vi "CRYAttack and Release.vi"(4 "Sine waves":T1(array[cluster]), 5 "Attack":sgl[](array[numeric]), 6 "Search range":string[](array[string]), 7 "% recovery":dbl=0.02 format="%.2f", 8 "All points":bool, 9 "Sampling rate":dbl format="%.2f", 10 "Attack? (T)":bool=TRUE, 11 "Data in":T2={"Name"="", "Curve"=[], "X data"=1, "Y data"=1, "Z data"=1, "X axis"=0, "Y axis"=1, "Z axis"=1, "X unit"="Hz", "Y unit"="", "Z unit"="deg.", "X dB ref"=1.0, "Y dB ref"=1.0, "Z dB ref"=1.0, "single val"=FALSE, "protected"=FALSE, "display X"=TRUE, "display Y"=TRUE, "display Z"=TRUE, "Test Info"="", "Step No."=0, "Plot Settings"={"Color"=0, "Interpolation"=0, "Point Style"=0, "Line Style"=0, "Point Color"=0, "Line Width"=0, "Bar Plot Style"=0, "Fill To"=0}, "AutoProtect"=FALSE} {"Z data" items=["dB", "Lin"]; "X data" items=["dB", "Lin"]; "Y data" items=["dB", "Lin"]; "Z dB ref" format="%.1f"; "Z axis" items=["Log", "Lin"]; "X dB ref" format="%.1f"; "X axis" items=["Log", "Lin"]; "Y axis" items=["Log", "Lin"]; "Y dB ref" format="%.1f"; "Curve"."z" format="%.2f"; "Curve"."y" format="%.2f"; "Curve"."x" format="%.2f"}) -> (1 "dy":dbl, 2 "Envelope":dbl[](array[numeric]) format="%.2f", 3 "Attack or release time":dbl format="%.2f")   [LabVIEW 2013]
uses:
  Typedef Control/CRYData Cluster.ctl
  <vilib>/Analysis/2dsp.llb/Decimate (single shot, DBL).vi
  <vilib>/Analysis/3filter.llb/Bessel Filter (DBL).vi
  <vilib>/Analysis/NI_AALPro.lvlib
  <vilib>/Analysis/NI_AALBase.lvlib
panel:
  out "dy 2":dbl
  out "Waveform Graph 2":waveform(dbl)(graph)
  out "Waveform Graph":waveform(dbl)(graph)
  in  "Discard cycles right":i32
  in  "search for attack/release starting point?":bool=TRUE
  in  "I donot know?":bool
  in  "BP filtering":bool=TRUE
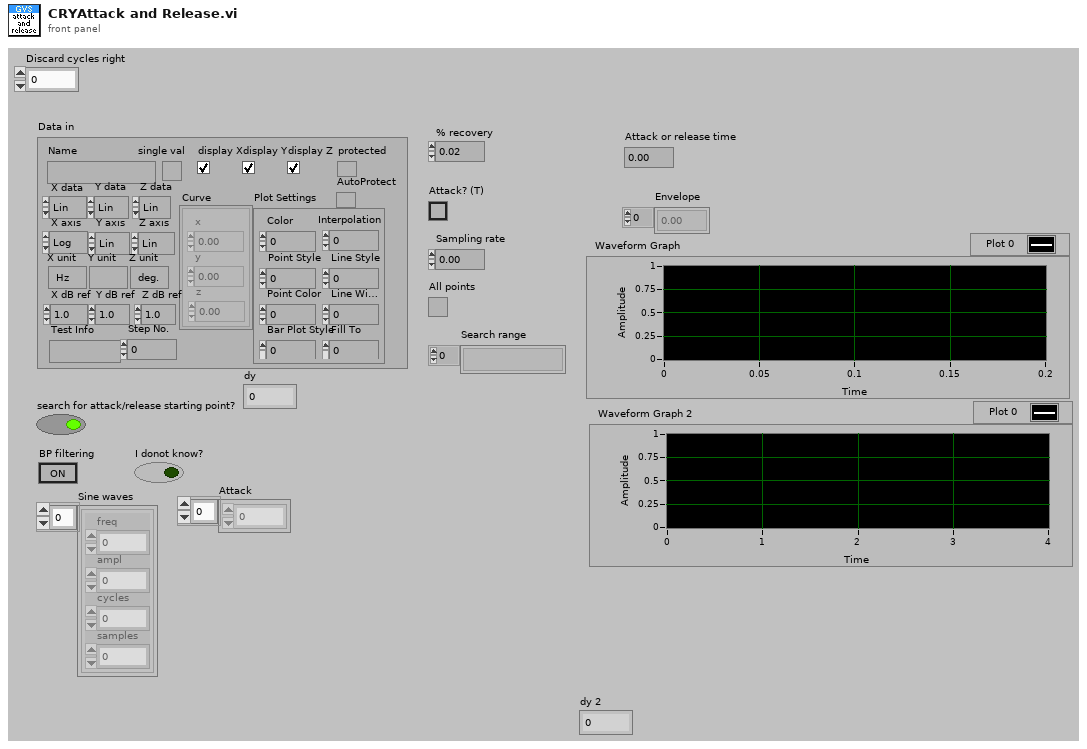
[diagram p1: front panel]
types:
  T1 = cluster{"freq":dbl, "ampl":dbl, "cycles":dbl, "samples":i32}[]
  T2 = typedef "CRYData Cluster.ctl" = cluster{"Name":string, "Curve":cluster{"x":dbl, "y":dbl, "z":dbl}[], "X data":u16, "Y data":u16, "Z data":u16, "X axis":u16, "Y axis":u16, "Z axis":u16, "X unit":string, "Y unit":string, "Z unit":string, "X dB ref":dbl, "Y dB ref":dbl, "Z dB ref":dbl, "single val":bool, "protected":bool, "display X":bool, "display Y":bool, "display Z":bool, "Test Info":string, "Step No.":i32, "Plot Settings":cluster{"Color":u32, "Interpolation":u8, "Point Style":u8, "Line Style":u8, "Point Color":u32, "Line Width":u8, "Bar Plot Style":u8, "Fill To":i16}, "AutoProtect":bool}
  T3 = cluster{"freq":dbl, "ampl":dbl, "cycles":dbl, "samples":i32}
  T4 = enum32{"Lowpass", "Highpass", "Bandpass", "Bandstop"}
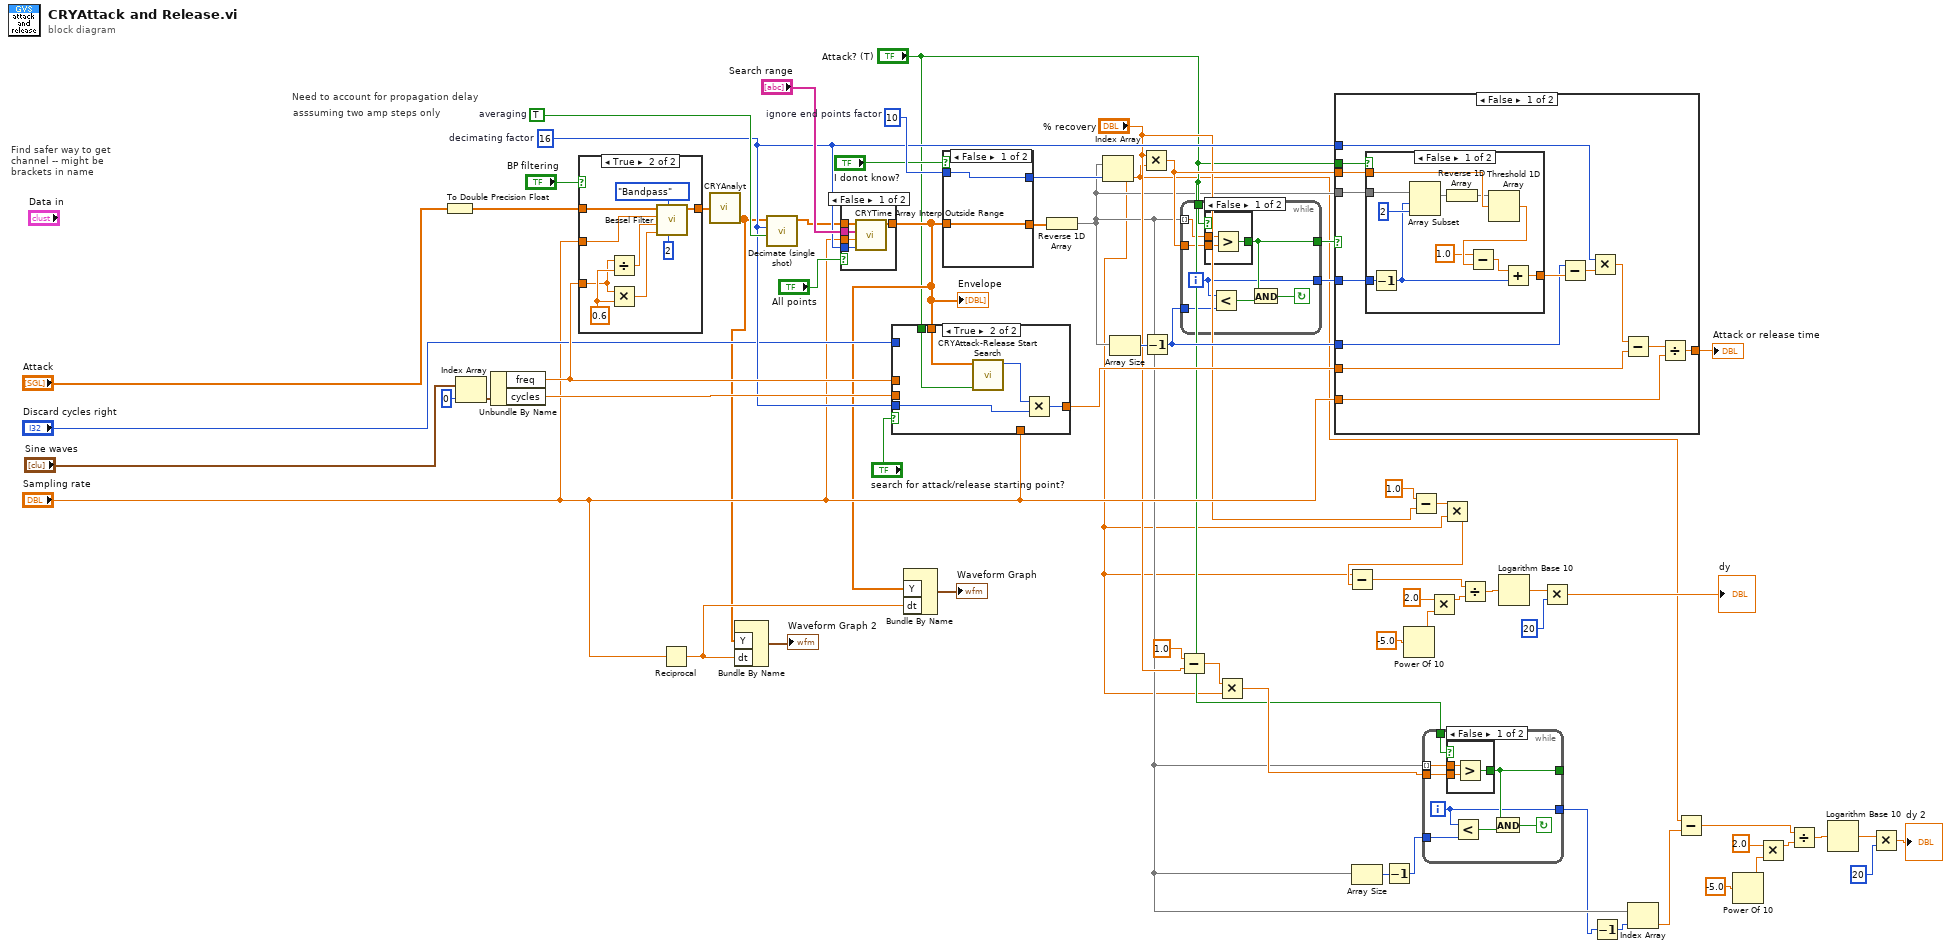
[diagram p0: block diagram]
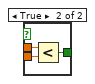
[diagram p2: hidden frame]
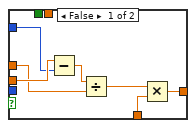
[diagram p3: hidden frame]
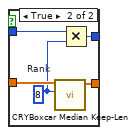
[diagram p5: hidden frame]
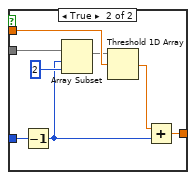
[diagram p7: hidden frame]
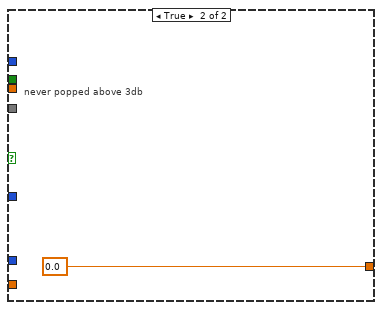
[diagram p8: hidden frame]
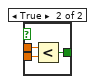
[diagram p9: hidden frame]
diagram:
  w57 = 10  # ignore end points factor
  w66 = TRUE  # averaging
  w48 = 16  # decimating factor
  # "Need to account for propagation delay"
  # "asssuming two amp steps only"
  # "Find safer way to get channel -- might be brackets in name"
  n1 = To Double Precision Float(number="Attack") -> (double precision float=w52:dbl[])
  n2 = Index Array(array="Sine waves", index=0 ("Index")) -> (element=w60:T3)
  n3 = Unbundle By Name(w60) -> ("freq"=w55:dbl, "cycles"=w56:dbl)
  n4 = case shown="True" "BP filtering" {
    tunnel: [w67 w76] -> w42
    tunnel: w52 -> [w67 w71]
    tunnel: w55 -> [_ w70]
    tunnel: "Sampling rate" -> [_ w69]
    frame False {
    }
    frame True {
      w75 = 0.6
      n5 = Divide(x=w70, y=w75) -> (x/y=w74:dbl)
      n6 = Multiply(x=w70, y=w75) -> (x*y=w73:dbl)
      n7 = call-poly <vilib>:"Bessel Filter.vi"("order"=2, "filter type"=T4."Bandpass", "low cutoff freq: fl"=w73, "high cutoff freq: fh"=w74, "sampling freq: fs"=w69, "X"=w71) -> ("Filtered X"=w76:dbl[])  [unwired: 1 in, 2 out]
    }
  }
  n8 = Reciprocal(x="Sampling rate") -> (1/x=w40:dbl)
  n9 = call "CRYAnalyt.vi"("Input"=w42) -> ("Magn"=w37:dbl[])  [unwired: 4 out]
  n10 = Bundle By Name("Y"=w37, "dt"=w40) -> (→"Waveform Graph 2":waveform(dbl))  [unwired: 1 in]
  n11 = call-poly <vilib>:"Decimate (single shot).vi"("averaging"=w66, "decimating factor"=w48, "X"=w37) -> ("Decimated Array"=w38:dbl[])  [unwired: 8 out]
  n12 = case shown="False" "All points" {
    tunnel: w38 -> [w81 w82]
    tunnel: [w80 w82] -> w41
    tunnel: "Search range" -> [w79 _]
    tunnel: "Sampling rate" -> [w78 _]
    tunnel: w48 -> [w77 _]
    frame False {
      n13 = call "CRYTime Array Interp Outside Range.vi"("Decimating factor"=w77, "Sampling rate"=w78, "Search range (ms)"=w79, "Points in time"=w81) -> ("Processed points in time"=w80:dbl[])  [unwired: 7 out]
    }
    frame True {
    }
  }
  "Envelope" <- w41
  n14 = case shown="True" "search for attack/release starting point?" {
    tunnel: [w88 w90] -> w59
    tunnel: w56 -> [w87 _]
    tunnel: "Discard cycles right" -> [w85 _]
    tunnel: w55 -> [w84 _]
    tunnel: "Sampling rate" -> [w83 _]
    tunnel: w41 -> [_ w94]
    tunnel: "Attack? (T)" -> [_ w93]
    tunnel: w48 -> [_ w92]
    frame False {
      n15 = Subtract(x=w87, y=w85) -> (x-y=w86:dbl)
      n16 = Divide(x=w86, y=w84) -> (x/y=w89:dbl)
      n17 = Multiply(x=w89, y=w83) -> (x*y=w88:dbl)
    }
    frame True {
      n18 = call "CRYAttack-Release Start Search.vi"("Attack? (T)"=w93, "Time data in"=w94) -> ("Pulse start index"=w91:i32)  [unwired: 2 in, 7 out]
      n19 = Multiply(x=w91, y=w92) -> (x*y=w90:i32)
    }
  }
  n20 = Bundle By Name("Y"=w41, "dt"=w40) -> (→"Waveform Graph":waveform(dbl))  [unwired: 1 in]
  n21 = case shown="False" "I donot know?" {
    tunnel: w41 -> [w96 w101]
    tunnel: [w96 w100] -> w58
    tunnel: w57 -> [w95 w98]
    tunnel: [w95 w97] -> w34
    frame False {
    }
    frame True {
      w99 = 8  # Rank
      n22 = call "CRYBoxcar Median Keep-Len.vi"("Rank"=w99, "Measured curve"=w101) -> ("Smoothed curve"=w100:dbl[])  [unwired: 9 out]
      n23 = Multiply(x=w98, y=w99) -> (x*y=w97:i32)
    }
  }
  n24 = Reverse 1D Array(array=w58) -> (reversed array=w13:dbl[])
  n25 = Index Array(array=w13, index=w34) -> (element=w1:dbl)
  n26 = Array Size(array=w13) -> (size(s)=w65:i32)
  n27 = Multiply(x="% recovery", y=w1) -> (x*y=w22:dbl)
  n28 = Decrement(x=w65) -> (x-1=w63:i32)
  n29 = Subtract(x=1.0, y="% recovery") -> (x-y=w16:dbl)
  n30 = while {
    tunnel: w13 -> [w107] mode=indexing
    tunnel: w63 -> [w109]
    tunnel: w22 -> [w108]
    tunnel: [w104] -> w64
    tunnel: [w103] -> w35
    tunnel: "Attack? (T)" -> [w102]
    i -> [w103]
    stop <- w105 continue-if-true
    n31 = case shown="False" w102 {
      tunnel: w108 -> [w111 w115]
      tunnel: w107 -> [w112 w114]
      tunnel: [w110 w113] -> w104
      frame False {
        n32 = Greater?(x=w112, y=w111) -> (0:w110:bool)
      }
      frame True {
        n33 = Less?(x=w114, y=w115) -> (x < y?=w113:bool)
      }
    }
    n34 = Less?(x=w103, y=w109) -> (x < y?=w106:bool)
    n35 = And(x=w104, y=w106) -> (x .and. y?=w105:bool)
  }
  n36 = Multiply(x=w16, y=w1) -> (x*y=w15:dbl)
  n37 = case shown="False" w64 {
    tunnel: w13 -> [w128 _]
    tunnel: w35 -> [w125 _]
    tunnel: w22 -> [w127 _]
    tunnel: w59 -> [w126 _]
    tunnel: w63 -> [w123 _]
    tunnel: "Sampling rate" -> [w122 _]
    tunnel: [w116 0.0] -> w62
    tunnel: w48 -> [w120 _]
    tunnel: "Attack? (T)" -> [w117 _]
    frame False {
      n38 = case shown="False" w117 {
        tunnel: w128 -> [w138 w146]
        tunnel: w127 -> [w137 w145]
        tunnel: w125 -> [w135 w143]
        tunnel: [w134 w141] -> w124
        frame False {
          n39 = Decrement(x=w135) -> (x-1=w133:i32)
          n40 = Array Subset(array=w138, index=w133, length=2 ("Array Length")) -> (w136:dbl[])
          n41 = Reverse 1D Array(array=w136) -> (reversed array=w132:dbl[])
          n42 = Threshold 1D Array(2:w137, 3:w132) -> (0:w131:dbl)  [unwired: 1 out]
          n43 = Subtract(x=1.0, y=w131) -> (x-y=w129:dbl)
          n44 = Add(x=w129, y=w133) -> (x+y=w134:dbl)
        }
        frame True {
          n45 = Decrement(x=w143) -> (x-1=w140:i32)
          n46 = Array Subset(array=w146, index=w140, length=2 ("Array Length")) -> (w144:dbl[])
          n47 = Threshold 1D Array(2:w145, 3:w144) -> (0:w142:dbl)  [unwired: 1 out]
          n48 = Add(x=w142, y=w140) -> (x+y=w141:dbl)
        }
      }
      n49 = Subtract(x=w123, y=w124) -> (x-y=w119:dbl)
      n50 = Multiply(x=w120, y=w119) -> (x*y=w118:dbl)
      n51 = Subtract(x=w118, y=w126) -> (x-y=w121:dbl)
      n52 = Divide(x=w121, y=w122) -> (x/y=w116:dbl)
    }
    frame True {
      # "never popped above 3db"
    }
  }
  "Attack or release time" <- w62
  n53 = Array Size(array=w13) -> (size(s)=w19:i32)
  n54 = Decrement(x=w19) -> (x-1=w20:i32)
  n55 = Power Of 10(x=-5.0) -> (10^x=w29:dbl)
  n56 = Subtract(x=1.0, y="% recovery") -> (x-y=w23:dbl)
  n57 = while {
    tunnel: w20 -> [w156]
    tunnel: w15 -> [w155]
    tunnel: [w152] -> _
    tunnel: [w151] -> w12
    tunnel: "Attack? (T)" -> [w150]
    tunnel: w13 -> [w149] mode=indexing
    i -> [w151]
    stop <- w153 continue-if-true
    n58 = case shown="False" w150 {
      tunnel: w155 -> [w158 w162]
      tunnel: w149 -> [w159 w161]
      tunnel: [w157 w160] -> w152
      frame False {
        n59 = Greater?(x=w159, y=w158) -> (0:w157:bool)
      }
      frame True {
        n60 = Less?(x=w161, y=w162) -> (x < y?=w160:bool)
      }
    }
    n61 = Less?(x=w151, y=w156) -> (x < y?=w154:bool)
    n62 = And(x=w152, y=w154) -> (x .and. y?=w153:bool)
  }
  n63 = Multiply(x=2.0, y=w29) -> (x*y=w28:dbl)
  n64 = Multiply(x=w23, y=w1) -> (x*y=w21:dbl)
  n65 = Subtract(x=w1, y=w21) -> (x-y=w27:dbl)
  n66 = Divide(x=w27, y=w28) -> (x/y=w26:dbl)
  n67 = Logarithm Base 10(1:w26) -> (0:w33:dbl)
  n68 = Multiply(x=w33, y=20) -> (x*y=→"dy":dbl)
  n69 = Decrement(x=w12) -> (x-1=w36:i32)
  n70 = Index Array(array=w13, index=w36) -> (element=w2:dbl)
  n71 = Subtract(x=w1, y=w2) -> (x-y=w9:dbl)
  n72 = Power Of 10(x=-5.0) -> (10^x=w7:dbl)
  n73 = Multiply(x=2.0, y=w7) -> (x*y=w8:dbl)
  n74 = Divide(x=w9, y=w8) -> (x/y=w10:dbl)
  n75 = Logarithm Base 10(1:w10) -> (0:w3:dbl)
  n76 = Multiply(x=w3, y=20) -> (x*y=→"dy 2":dbl)
